vi "AgPSA _Read Trace (Swept SA) (bytes override).vi"(7 "byte count":u32=100000, 8 "error in (no error)":errorcluster, 9 "Trace Name (1: Trace 1)":i32(ring)=1 items=["Trace 1"=1, "Trace 2"=2, "Trace 3"=3, "Trace 4"=4], 10 "Timeout (10000 ms)":i32=10000 format="%.0g", 11 "VISA resource name":refnum<visa-resource-name>) -> (0 "error out":errorcluster, 2 "Trace Waveform":cluster{"X Array":dbl[], "Y Array":dbl[]}(graph), 3 "VISA resource name out":refnum<visa-resource-name>)   [LabVIEW 2015]
doc: "Reads the trace from the spectrum analyzer(Swept SA)."
uses:
  <instrlib>/Agilent MXA Series/Agilent MXA Series.lvlib
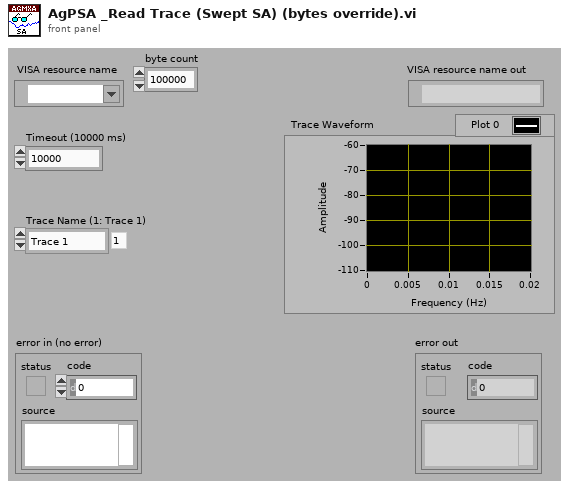
[diagram p1: front panel]
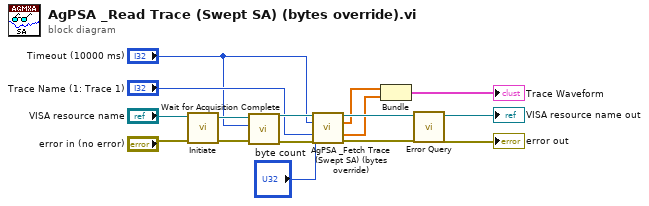
[diagram p0: block diagram]
diagram:
  n1 = call <instrlib>:"Initiate.vi"("error in (no error)"="error in (no error)", "VISA resource name"="VISA resource name") -> ("error out"=w13:errorcluster, "VISA resource name out"=w14:refnum<visa-resource-name>)  [unwired: 8 in]
  n2 = call <instrlib>:"Wait for Acquisition Complete.vi"("error in (no error)"=w13, "Maximum Time (10000)"="Timeout (10000 ms)", "VISA resource name"=w14) -> ("error out"=w11:errorcluster, "VISA resource name out"=w12:refnum<visa-resource-name>)  [unwired: 7 in]
  n3 = call "AgPSA _Fetch Trace (Swept SA) (bytes override).vi"("VISA resource name"=w12, "Timeout (10000 ms)"="Timeout (10000 ms)", "byte count"="byte count", "Trace Name (1: Trace 1)"="Trace Name (1: Trace 1)", "error in (no error)"=w11) -> ("VISA resource name out"=w9:refnum<visa-resource-name>, "X Array"=w5:dbl[], "Y Array"=w4:dbl[], "error out"=w8:errorcluster)  [unwired: 7 in]
  n4 = Bundle("X Array"=w5, "Y Array"=w4) -> (→"Trace Waveform":cluster{"X Array":dbl[], "Y Array":dbl[]})  [unwired: 1 in]
  n5 = call <instrlib>:"Error Query.vi"("error in (no error)"=w8, "VISA resource name"=w9) -> ("error out"=→"error out":errorcluster, "VISA resource name out"=→"VISA resource name out":refnum<visa-resource-name>)  [unwired: 6 in, 2 out]
